vi "Teleop.vi"(10 "Match Info":T1={"Autonomous Elapsed Seconds"=0.0, "TeleOp Elapsed Seconds"=0.0, "Disabled Elapsed Seconds"=0.0, "Visited Autonomous"=FALSE, "Visited TeleOp"=FALSE, "Visited Disabled"=FALSE, "Autonomous Settings"={"Autonomous Style"=enum."Independent", "VI Refnum"=refnum}}, 11 "Call Context":T2) -> ()   [LabVIEW 2016]
doc: "This VI is called for each TeleOp packet received from the DS where the robot is not disabled. It is often used to read from the joysticks and update I/O or to update setpoints for timed control loops. It should complete and return within 20 milliseconds or it may miss DS packets."
uses:
  <vilib>/Rock Robotics/WPI/DriverStation/WPI_DriverStationDerivedRobotMode.ctl
  <vilib>/Rock Robotics/WPI/DriverStation/WPI_DriverStationMatch Info.ctl
  <vilib>/Rock Robotics/WPI/Solenoid/WPI_SolenoidValue.ctl
  <vilib>/Rock Robotics/Network Tables/NT Read Boolean.vi
  <vilib>/Rock Robotics/Network Tables/NT Read Number.vi
  <vilib>/Rock Robotics/WPI/Utilities/WPI_GetSetVariantRefNum.vi
  <vilib>/Rock Robotics/WPI/Joystick/WPI_JoystickArcadeMapping.vi
panel:
  in  "Boolean":bool=TRUE
  out "Sample Slider 0":dbl(slide) scale=0.0..5.0
  out "Sample Boolean 1":bool
  out "Sample Boolean 0":bool
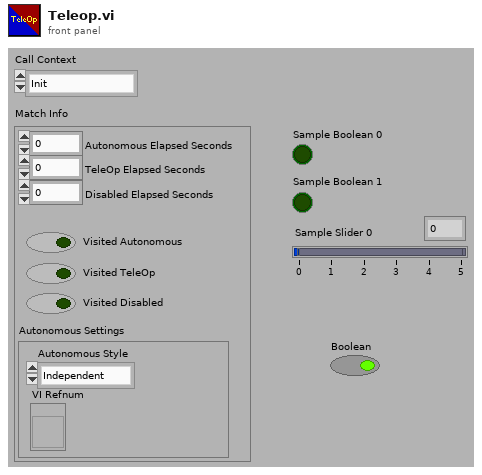
[diagram p1: front panel]
types:
  T1 = typedef "WPI_DriverStationMatch Info.ctl" = cluster{"Autonomous Elapsed Seconds":dbl, "TeleOp Elapsed Seconds":dbl, "Disabled Elapsed Seconds":dbl, "Visited Autonomous":bool, "Visited TeleOp":bool, "Visited Disabled":bool, "Autonomous Settings":cluster{"Autonomous Style":enum16{"Iterative", "Independent"}, "VI Refnum":refnum<vi>}}
  T2 = typedef "WPI_DriverStationDerivedRobotMode.ctl" = enum16{"Init", "Execute", "Stop"}
  T3 = typedef "WPI_JoystickDevRef.ctl" = cluster{"Device":T4}
  T4 = typedef "WPI_JoystickDeviceEnum.ctl" = enum16{"USB 0", "USB 1", "USB 2", "USB 3", "USB 4", "USB 5"}
  T5 = cluster{"Gyro":string, "Mtr 1":string, "Mtr 2":string}
  T6 = typedef "WPI_SolenoidValue.ctl" = enum16{"Off", "On", "Forward", "Reverse"}
  T7 = typedef "WPI_SolenoidDevRef.ctl" = cluster{"DevStatus":errorcluster, "Pneumatics Control Module":u8, "Forward Solenoid Channel":T8, "Reverse Solenoid Channel":T8}
  T8 = typedef "WPI_SolenoidChannel.ctl" = enum8{"Solenoid 0", "Solenoid 1", "Solenoid 2", "Solenoid 3", "Solenoid 4", "Solenoid 5", "Solenoid 6", "Solenoid 7", "Invalid"}
  T9 = typedef "WPI_MotorControlDeviceRef.ctl" = cluster{"DeviceStatus":errorcluster, "Type":T10, "PWM":cluster{"PWM Channel":T11, "DeadBand":T12}, "CAN":cluster{"Device Number":u8, "SetOutput VI Ref":variant, "GetOutput VI Ref":variant, "Enable VI Ref":variant, "Disable VI Ref":variant, "Data":variant}, "Invert":bool}
  T10 = typedef "WPI_MotorControlType.ctl" = enum16{"PWM", "CAN"}
  T11 = typedef "FPGA_DIOPWMChannel.ctl" = enum8{"PWM 0", "PWM 1", "PWM 2", "PWM 3", "PWM 4", "PWM 5", "PWM 6", "PWM 7", "PWM 8", "PWM 9", "PWM MXP 0", "PWM MXP 1", "PWM MXP 2", "PWM MXP 3", "PWM MXP 4", "PWM MXP 5", "PWM MXP 6", "PWM MXP 7", "PWM MXP 8", "PWM MXP 9", "Invalid"}
  T12 = typedef "WPI_PWMDeadband.ctl" = cluster{"Name":string, "maxPositivePwm":i32, "minPositivePwm":i32, "centerPwm":i32, "maxNegativePwm":i32, "minNegativePwm":i32, "angularRange":u16}
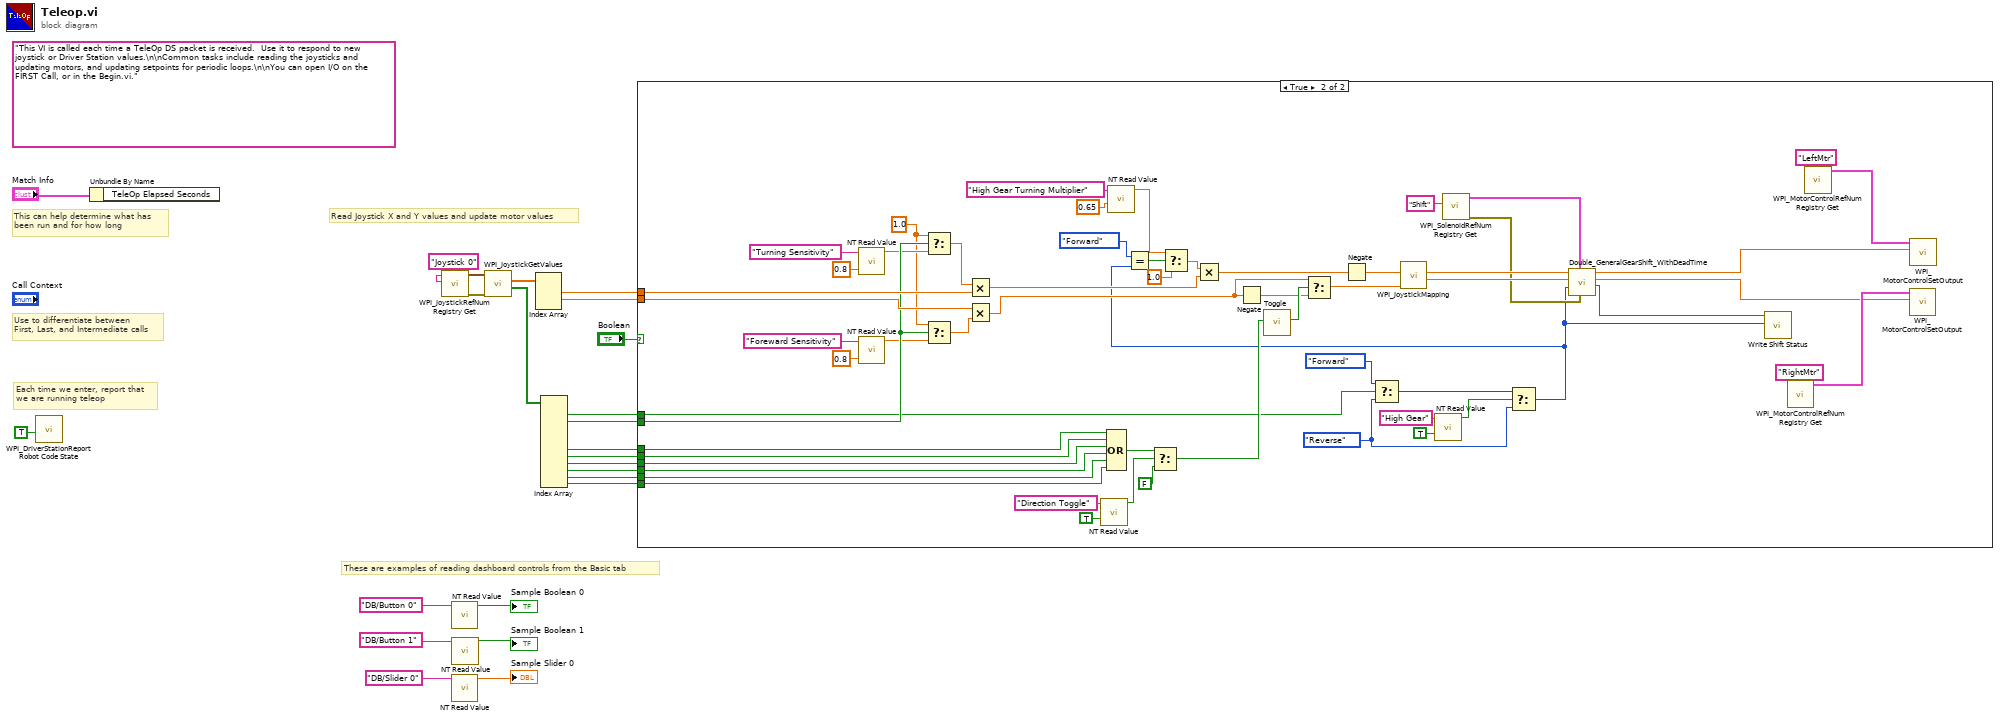
[diagram p0: block diagram]
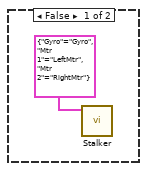
[diagram p2: hidden frame]
diagram:
  (unwired) "This VI is called each time a TeleOp DS packet is received.  Use it to respond to new joystick or Driver Station values.\n\nCommon tasks include reading the joysticks and updating motors, and updating setpoints for periodic loops.\n\nYou can open I/O on the FIRST Call, or in the Begin.vi."
  # "These are examples of reading dashboard controls from the Basic tab"
  # "Each time we enter, report that\nwe are running teleop"
  # "Use to differentiate between\nFirst, Last, and Intermediate calls"
  # "This can help determine what has\nbeen run and for how long"
  # "Read Joystick X and Y values and update motor values"
  n1 = call <vilib>:"WPI_DriverStationReport Robot Code State.vi"("TeleOp"=TRUE ("Autonomous")) -> ()  [unwired: 10 in, 1 out]
  n2 = Unbundle By Name("Match Info") -> ()  [unwired: 1 out]
  n3 = call <vilib>:"WPI_JoystickRefNum Registry Get.vi"("refnum name"="Joystick 0") -> ("error out"=w13:errorcluster, "JoystickDevRef"=w16:T3)  [unwired: 1 in, 8 out]
  n4 = call-poly <vilib>:"NT Read Value.vi"("Name"="DB/Button 0" ("refnum name")) -> ("Boolean"=→"Sample Boolean 0":bool)  [unwired: 9 in, 1 out]
  n5 = call-poly <vilib>:"NT Read Value.vi"("Name"="DB/Slider 0" ("refnum name")) -> ("Numeric"=→"Sample Slider 0":dbl)  [unwired: 9 in, 1 out]
  n6 = call-poly <vilib>:"NT Read Value.vi"("Name"="DB/Button 1" ("refnum name")) -> ("Boolean"=→"Sample Boolean 1":bool)  [unwired: 9 in, 1 out]
  n7 = call <vilib>:"WPI_JoystickGetValues.vi"("error in (no error)"=w13, "JoystickDevRef"=w16) -> ("Buttons"=w14:bool[], "Axes"=w15:dbl[])  [unwired: 5 in, 3 out]
  n8 = Index Array(array=w15) -> (element #1=w5:dbl, element #2=w4:dbl)  [unwired: 3 in, 1 out]
  n9 = Index Array(array=w14) -> (element #1=w6:bool, element #2=w3:bool, element #6=w12:bool, element #7=w11:bool, element #8=w10:bool, element #9=w9:bool, element #10=w7:bool, element #11=w8:bool)  [unwired: 11 in, 3 out]
  n10 = case shown="True" "Boolean" {
    tunnel: w12 -> [_ w83]
    tunnel: w11 -> [_ w82]
    tunnel: w10 -> [_ w81]
    tunnel: w9 -> [_ w80]
    tunnel: w8 -> [_ w79]
    tunnel: w7 -> [_ w78]
    tunnel: w6 -> [_ w32]
    tunnel: w5 -> [_ w70]
    tunnel: w4 -> [_ w69]
    tunnel: w3 -> [_ w68]
    frame False {
      n11 = call "Stalker.vi"("Refnum's In"=T5 {"Gyro"="Gyro", "Mtr 1"="LeftMtr", "Mtr 2"="RightMtr"}) -> ()  [unwired: 9 in, 2 out]
    }
    frame True {
      w36 = 1.0 ("t")
      w26 = WPI_SolenoidValue."Reverse" ("Shift Value")
      n12 = call-poly <vilib>:"NT Read Value.vi"("Default Value"=0.8, "Name"="Turning Sensitivity") -> ("Numeric"=w38:dbl)  [unwired: 8 in, 1 out]
      n13 = call-poly <vilib>:"NT Read Value.vi"("Default Value"=0.8, "Name"="Foreward Sensitivity") -> ("Numeric"=w40:dbl)  [unwired: 8 in, 1 out]
      n14 = Select(t=w36, s=w68, f=w38) -> (s? t:f=w37:dbl)
      n15 = Select(t=w36, s=w68, f=w40) -> (s? t:f=w39:dbl)
      n16 = Multiply(x=w37, y=w70) -> (x*y=w41:dbl)
      n17 = Multiply(x=w69, y=w39) -> (x*y=w42:dbl)
      n18 = call-poly <vilib>:"NT Read Value.vi"("Default Value"=TRUE, "Name"="Direction Toggle") -> ("Boolean"=w53:bool)  [unwired: 8 in, 1 out]
      n19 = Compound Arithmetic op=OR(w83, w82, w81, w80, w78, w79) -> (w54:bool)
      n20 = call-poly <vilib>:"NT Read Value.vi"("Default Value"=0.65, "Name"="High Gear Turning Multiplier") -> ("Numeric"=w48:dbl)  [unwired: 8 in, 1 out]
      n21 = Select(t=w54, s=w53, f=FALSE) -> (s? t:f=w50:bool)
      n22 = Negate(x=w42) -> (-x=w66:dbl)
      n23 = call "Toggle.vi"("Input"=w50) -> ("Output"=w67:bool)  [unwired: 10 in]
      n24 = Select(t=w42, s=w67, f=w66) -> (s? t:f=w35:dbl)
      n25 = Select(t=WPI_SolenoidValue."Forward" ("Shift Value"), s=w32, f=w26) -> (s? t:f=w28:T6)
      n26 = call-poly <vilib>:"NT Read Value.vi"("Default Value"=TRUE, "Name"="High Gear") -> ("Boolean"=w27:bool)  [unwired: 8 in, 1 out]
      n27 = call <vilib>:"WPI_SolenoidRefNum Registry Get.vi"("refnum name"="Shift") -> ("error out"=w60:errorcluster, "SolenoidDevRef"=w61:T7)  [unwired: 9 in]
      n28 = Select(t=w28, s=w27, f=w26) -> (s? t:f=w29:T6)
      n29 = Equal?(x=WPI_SolenoidValue."Forward" ("Shift Value"), y=w29) -> (x = y?=w59:bool)
      n30 = Select(t=w48, s=w59, f=1.0) -> (s? t:f=w56:dbl)
      n31 = Multiply(x=w56, y=w41) -> (x*y=w34:dbl)
      n32 = Negate(x=w34) -> (-x=w33:dbl)
      n33 = call-poly <vilib>:"WPI_JoystickMapping.vi"("Y axis value"=w35, "X axis value"=w33) -> ("Right Motor Value"=w64:dbl, "Left Motor Value"=w65:dbl)  [unwired: 8 in]
      n34 = call "Double_GeneralGearShift_WithDeadTime.vi"("error In"=w60, "ShifterRef"=w61, "Shift Value"=w29, "Right"=w64, "Left"=w65) -> ("Shifting"=w71:bool, "Right Output"=w72:dbl, "Left Output"=w73:dbl)  [unwired: 3 in, 1 out]
      n35 = call "Write Shift Status.vi"("Gear"=w29, "Output"=w71) -> ()  [unwired: 9 in, 1 out]
      n36 = call <vilib>:"WPI_MotorControlRefNum Registry Get.vi"("refnum name"="RightMtr") -> ("MotorControlDevRef"=w76:T9)  [unwired: 9 in, 1 out]
      n37 = call <vilib>:"WPI_MotorControlRefNum Registry Get.vi"("refnum name"="LeftMtr") -> ("MotorControlDevRef"=w77:T9)  [unwired: 9 in, 1 out]
      n38 = call <vilib>:"WPI_MotorControlSetOutput.vi"("Output"=w72, "MotorControlDevRef"=w76) -> ()  [unwired: 7 in, 3 out]
      n39 = call <vilib>:"WPI_MotorControlSetOutput.vi"("Output"=w73, "MotorControlDevRef"=w77) -> ()  [unwired: 7 in, 3 out]
    }
  }
